vi "WPI_DigitalModulePulse.vi"(8 "error in (no error)":errorcluster, 9 "PulseLength":u8 format="%0d", 10 "DIOChannel":T1=enum."DIO 1", 11 "DigitalModuleDevRef":T2) -> (0 "error out":errorcluster, 3 "DigitalModuleDevRef":T2)   [LabVIEW 2017]
doc: "This software is licensed. Open the labview\\readme\\WPI Robotics Library Open Source License.txt file for more information."
uses:
  <vilib>/Rock Robotics/WPI/DigitalModule/WPI_DigitalModuleDeviceRef.ctl
  <vilib>/Rock Robotics/SystemInterfaces/DIO/FPGA_DIOChannel.ctl
  <vilib>/Rock Robotics/SystemInterfaces/System/FPGA_SystemGet.vi
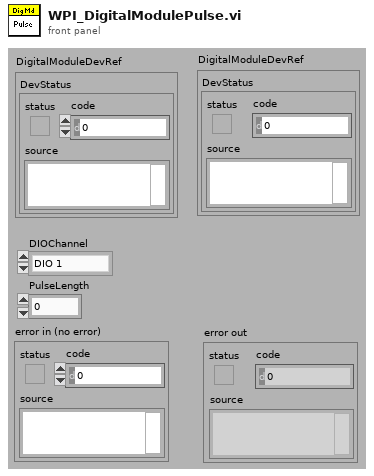
[diagram p1: front panel]
types:
  T1 = typedef "FPGA_DIOChannel.ctl" = enum8{"DIO 0", "DIO 1", "DIO 2", "DIO 3", "DIO 4", "DIO 5", "DIO 6", "DIO 7", "DIO 8", "DIO 9", "DIO MXP 0", "DIO MXP 1", "DIO MXP 2", "DIO MXP 3", "DIO MXP 4", "DIO MXP 5", "DIO MXP 6", "DIO MXP 7", "DIO MXP 8", "DIO MXP 9", "DIO MXP 10", "DIO MXP 11", "DIO MXP 12", "DIO MXP 13", "DIO MXP 14", "DIO MXP 15", "SPI Port CS1", "SPI Port CS2", "SPI Port CS3", "SPI Port MISO", "SPI Port MOSI", "Invalid"}
  T2 = typedef "WPI_DigitalModuleDeviceRef.ctl" = cluster{"DevStatus":errorcluster}
  T3 = typedef "FPGA_DIODevRef.ctl" = cluster{"DevStatus":errorcluster}
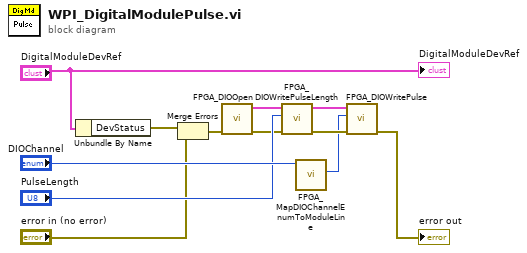
[diagram p0: block diagram]
diagram:
  n1 = Unbundle By Name("DigitalModuleDevRef") -> ("DevStatus"=w4:errorcluster)
  n2 = Merge Errors(w4, "error in (no error)") -> (w3:errorcluster)
  n3 = call <vilib>:"FPGA_DIOOpen.vi"("error in (no error)"=w3) -> ("error out"=w9:errorcluster, "DIODeviceRef"=w8:T3)  [unwired: 1 in, 8 out]
  n4 = call <vilib>:"FPGA_DIOWritePulseLength.vi"("error in (no error)"=w9, "PulseLength"="PulseLength", "DIODeviceRef"=w8) -> ("error out"=w6:errorcluster, "DIODeviceRef"=w7:T3)  [unwired: 7 out]
  n5 = call <vilib>:"FPGA_MapDIOChannelEnumToModuleLine.vi"("DIOChannel"="DIOChannel") -> ("ActualDIOBitMask(U32)"=w5:u32)  [unwired: 10 out]
  n6 = call <vilib>:"FPGA_DIOWritePulse.vi"("error in (no error)"=w6, "Pulse"=w5, "DIODeviceRef"=w7) -> ("error out"=→"error out":errorcluster)  [unwired: 8 out]
  "DigitalModuleDevRef" <- "DigitalModuleDevRef"
